vi "Actor Core.vi"(8 "error in":errorcluster, 11 "Controller in":refnum<class "Controller.lvclass">) -> (0 "error out":errorcluster, 3 "Actor out":refnum<class "Actor.lvclass">)   [LabVIEW 2014, in "Controller.lvlib" / "Controller.lvclass"]
doc: "(<B>Filename</B>: Actor Framework.lvlib:Actor.lvclass:Actor Core.vi)\n\nReceives messages to the actor, reacts to them, and initiates any error handling that may shut the actor down.\n\nDescendant classes may override this VI to append parallel tasks for the actor to complete while it handles messages. Overrides use the Call Parent Method node."
uses:
  Controller.lvclass
  <vilib>/ActorFramework/Actor/Actor.lvclass
  Data/xData.lvclass
  reusable/Data/Data.lvclass/Data.ctl
  Messages/Purge Switch Message/Purge Switch MSG.lvclass
  Messages/Update Switch State MSG/Update Switch MSG.lvclass/Update Switch MSG.ctl
  Calibration/O3 Frequency Train Actor/O3 Frequency Train Actor.lvclass
  <vilib>/ActorFramework/Actor/Actor.lvclass/Actor.ctl
  <vilib>/ActorFramework/Message Enqueuer/Message Enqueuer.lvclass/Message Enqueuer.ctl
  reusable/Data/Write Data ID.vi
  Messages/Update Switch State MSG/Write SwitchState.vi
  <vilib>/ActorFramework/Message Enqueuer/Init from Existing Queue.vi
  <vilib>/ActorFramework/Message Priority Queue/Priority Enqueue.vi
  <vilib>/ActorFramework/Message Enqueuer/Message Enqueuer.lvclass
  SuperActor/Ex Nested.lvclass
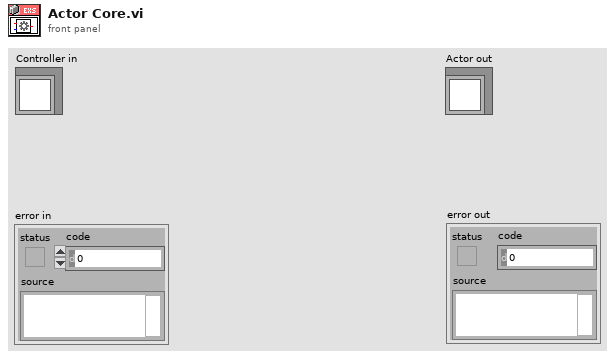
[diagram p1: front panel]
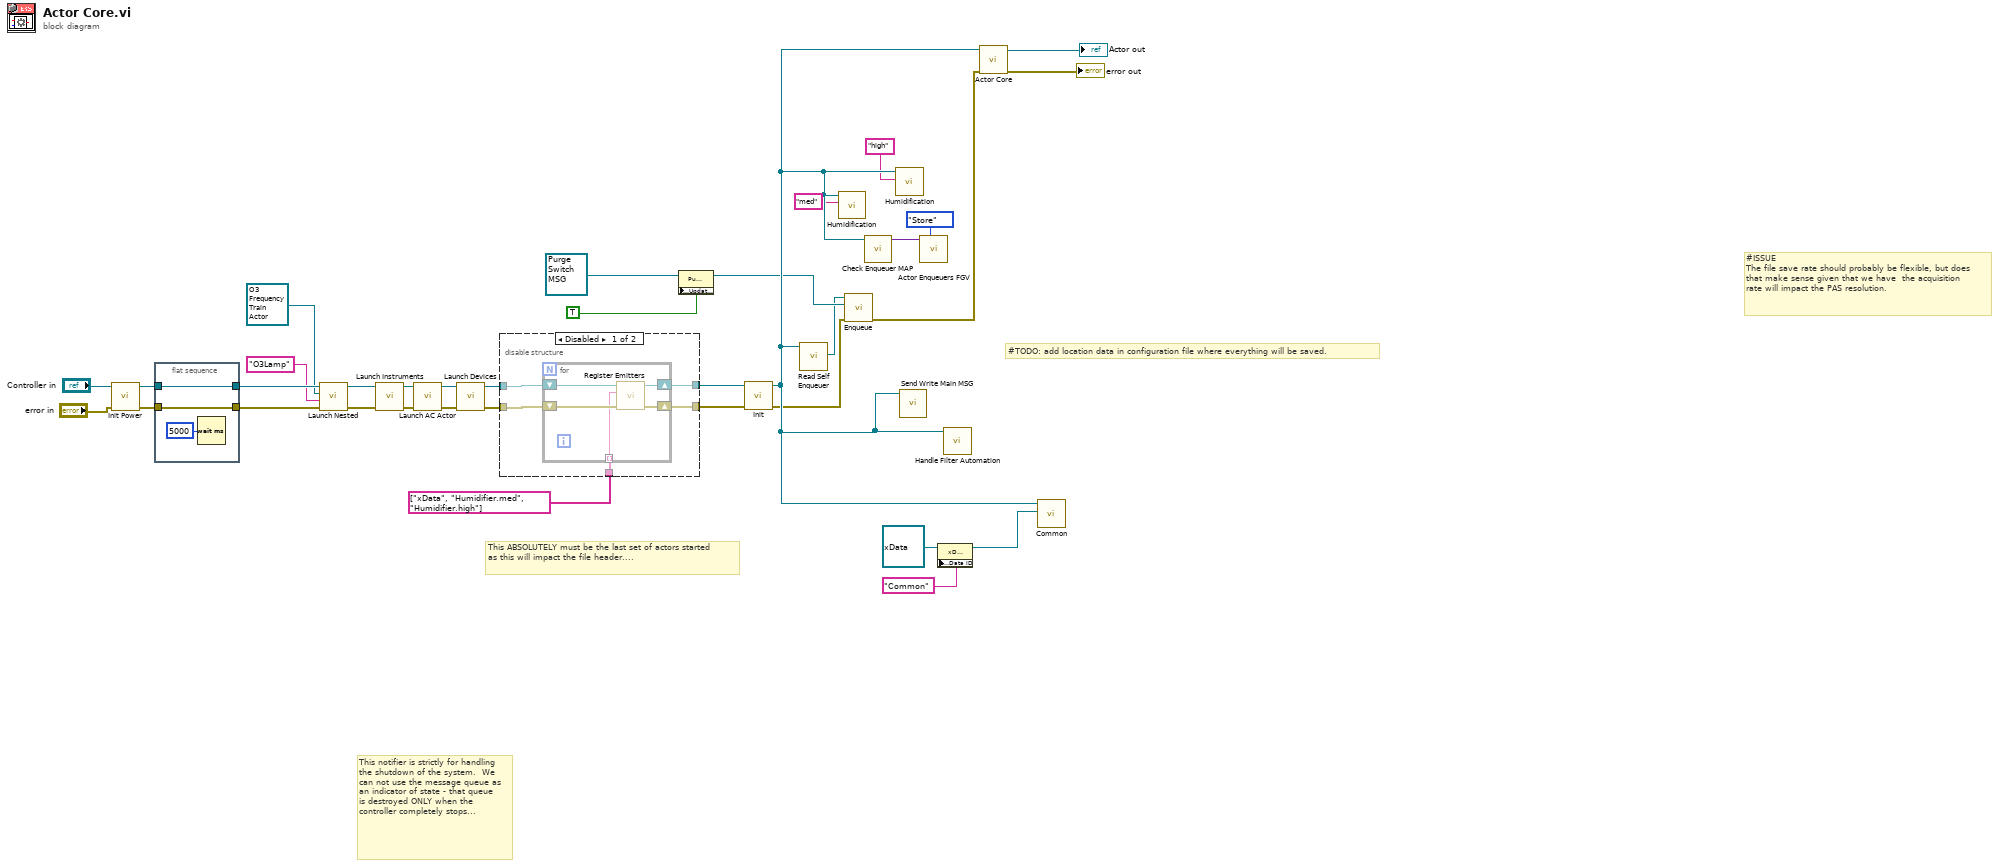
[diagram p0: block diagram]
diagram:
  # "This ABSOLUTELY must be the last set of actors started as this will impact the file header...."
  # "#TODO: add location data in configuration file where everything will be saved."
  # "This notifier is strictly for handling the shutdown of the system.  We can not use the message queue as an indicator of state - that queue is destroyed ONLY when the controller completely stops..."
  # "#ISSUE\nThe file save rate should probably be flexible, but does that make sense given that we have  the acquisition rate will impact the PAS resolution."
  n1 = call "Init Power.vi"("error in"="error in", "Controller in"="Controller in") -> ("error out"=w10:errorcluster, "Controller out"=w11:refnum<class "Controller.lvclass">)  [unwired: 8 in]
  n2 = flat-sequence {
    tunnel: [w37] -> w8
    tunnel: w11 -> [w37]
    tunnel: [w36] -> w7
    tunnel: w10 -> [w36]
    frame #0 {
      n3 = Wait (ms)(milliseconds to wait=u32 5000) -> ()  [unwired: 1 out]
    }
  }
  n4 = call "Launch Nested.vi"("Error In"=w7, "ID"="O3Lamp", "Nested Actor"=refnum<class "O3 Frequency Train Actor.lvclass"> refnum ("Calibration.lvlib:O3 Frequency Train Actors"), "Controller in"=w8) -> ("Error Out"=w6:errorcluster, "Controller out"=w9:refnum<class "Controller.lvclass">)  [unwired: 5 in, 1 out]
  n5 = call "Launch Instruments.vi"("error in"=w6, "Controller in"=w9) -> ("error out"=w22:errorcluster, "Controller out"=w21:refnum<class "Controller.lvclass">)  [unwired: 8 in]
  n6 = call "Launch AC Actor.vi"("error in"=w22, "Controller in"=w21) -> ("error out"=w20:errorcluster, "Controller out"=w17:refnum<class "Controller.lvclass">)  [unwired: 8 in]
  n7 = call "Launch Devices.vi"("error in"=w20, "Controller In"=w17) -> ("error out"=w19:errorcluster, "Controller Out"=w18:refnum<class "Controller.lvclass">)  [unwired: 8 in]
  n8 = disable-structure shown="Disabled" {
    disable-tunnel: w19 -> [w43 w49]
    disable-tunnel: w18 -> [w42 w50]
    disable-tunnel: [w41 w50] -> w13
    disable-tunnel: [w40 w49] -> w12
    disable-tunnel: string[] ["xData", "Humidifier.med", "Humidifier.high"] -> [w39 _]
    frame Disabled {
      n9 = for {
        shift-right: [w48] -> w40
        shift-left: w43 -> [w46]
        shift-right: [w47] -> w41
        shift-left: w42 -> [w45]
        tunnel: w39 -> [w44] mode=indexing
        n10 = call "Register Emitters.vi"("error in"=w46, "Emitter"=w44, "Controller in"=w45) -> ("error out"=w48:errorcluster, "Controller out"=w47:refnum<class "Controller.lvclass">)  [unwired: 7 in]
      }
    }
    frame Enabled {
    }
  }
  n11 = property class="Purge Switch"(reference=refnum<class "Purge Switch MSG.lvclass"> refnum ("Controller.lvlib:Purge Switch"), "Accessors:UpdateSw"=TRUE ("MFC_")) -> (reference out=w28:refnum<class "Purge Switch MSG.lvclass">)  [unwired: 1 in, 1 out]
  n12 = call "Init.vi"("error in"=w12, "Controller in"=w13) -> ("error out"=w29:errorcluster, "Controller out"=w30:refnum<class "Controller.lvclass">)  [unwired: 8 in]
  n13 = call <vilib>:"Read Self Enqueuer.vi"("Actor"=w30) -> ("Self Enqueuer"=w16:refnum<class "Message Enqueuer.lvclass">)  [unwired: 10 in]
  n14 = call "Humidification.vi"("Humidifier"="med", "Controller in"=w30) -> ()  [unwired: 10 in]
  n15 = call <vilib>:"Enqueue.vi"("error in (no error)"=w29, "Message"=w28, "Message Enqueuer in"=w16) -> ("error out"=w33:errorcluster)  [unwired: 7 in, 1 out]
  n16 = call "Check Enqueuer MAP.vi"("Controller in"=w30) -> ("Enqueuer Map"=w15:variant)  [unwired: 10 in]
  n17 = call "Humidification.vi"("Humidifier"="high", "Controller in"=w30) -> ()  [unwired: 10 in]
  n18 = call "Send Write Main MSG.vi"("Controller in"=w30) -> ()  [unwired: 11 in]
  n19 = call "Actor Enqueuers FGV.vi"("State"=enum16{"Store", "Send MSG"}."Store", "Enqueuer Map"=w15) -> ()  [unwired: 9 in, 1 out]
  n20 = property class="xData"(reference=refnum<class "xData.lvclass"> refnum ("xData.lvclass"), "Accessors:Data ID"="Common" ("Data ID")) -> (reference out=w25:refnum<class "xData.lvclass">)  [unwired: 1 in, 1 out]
  n21 = call "Handle Filter Automation.vi"("Controller in"=w30) -> ()  [unwired: 11 in]
  n22 = call-parent "Actor Core.vi"("error in"=w33, "Actor in"=w30) -> ("error out"=→"error out":errorcluster, "Actor out"=→"Actor out":refnum<class "Actor.lvclass">)  [unwired: 8 in]
  n23 = call "Common.vi"("xData in"=w25, "Controller in"=w30) -> ()  [unwired: 10 in]
